vi "SQLite Get Sequence.vi"(8 "error in (no error)":errorcluster, 11 "Main":string="0") -> (0 "error out":errorcluster, 1 "TestMode List":string[](array[string]), 2 "GetRowHeaderList":string[](array[string]), 3 "TestSequence":string[][](array[string]), 4 "VariableName List":string[](array[string]))   [LabVIEW 2017, in "SQLite.lvclass"]
doc: "get test sequence table.\n2016-09-07 15:47:21\nBy：蒋松\nEmail：jiangsong@outlook.com\nSina: @sushu1051"
uses:
  SQLite.lvclass
  SQLiteFileName.ctl
  TabelFullName.ctl
  <vilib>/Utility/error.llb/Trim Whitespace.vi
  <userlib>/_OpenG.lib/array/array.llb/Remove Duplicates from 1D Array (String)__ogtk.vi
  <userlib>/LabSQL/LabSQL.lvlib
  <userlib>/sushu/sushu.lvlib
panel:
  out "Select SQL CMD":string
  out "Array 2":string[](array[string])
  out "Result Set":string[][](table) caption="Result Set (from first statement with results)"
  out "Array":string[](array[string])
  in  "SequenceNum":string
  in  "Items":string
  in  "Sequence Value":T1
  # "insert 之前要先backup原有的数据，使Items在对应条目的最大值+1\n2015-11-03 16:45:40\nBy：蒋松\nEmail：jiangsong@outlook.com\nSina: @sushu1051"
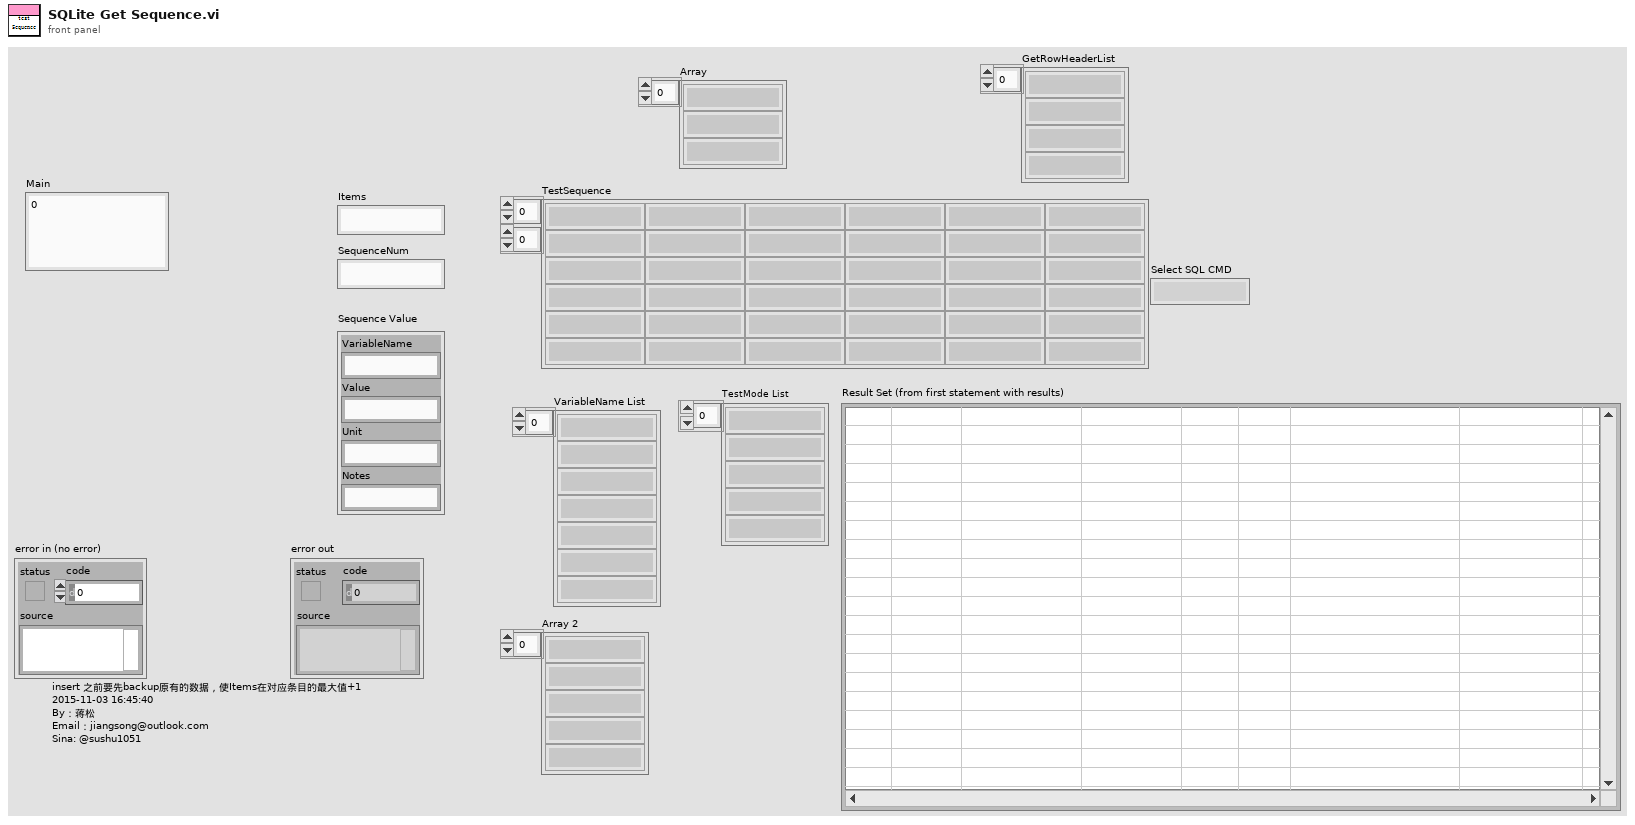
[diagram p1: front panel]
types:
  T1 = cluster{"VariableName":string, "Value":string, "Unit":string, "Notes":string}
  T2 = typedef "SQLite.lvclass/TabelFullName.ctl" = string
  T3 = typedef "SQLite.lvclass/SQLiteFileName.ctl" = string
  T4 = enum32{"invalid app kind", "Development System", "Run Time System", "Student Edition", "Embedded LabVIEW", "Evaluation", "Custom"}
  T5 = enum32{"Invalid", "Standard", "Closed", "Hidden", "Minimized", "Maximized"}
  T6 = enum16{"Other", "SQL2008", "SQLite", "Access", "MySQL"}
  T7 = cluster{"Core":cluster{"Current VI Reference":refnum<vi>, "Close Panel on Exit?":bool}}
  T8 = cluster{"Current VI Reference":refnum<vi>, "Close Panel on Exit?":bool}
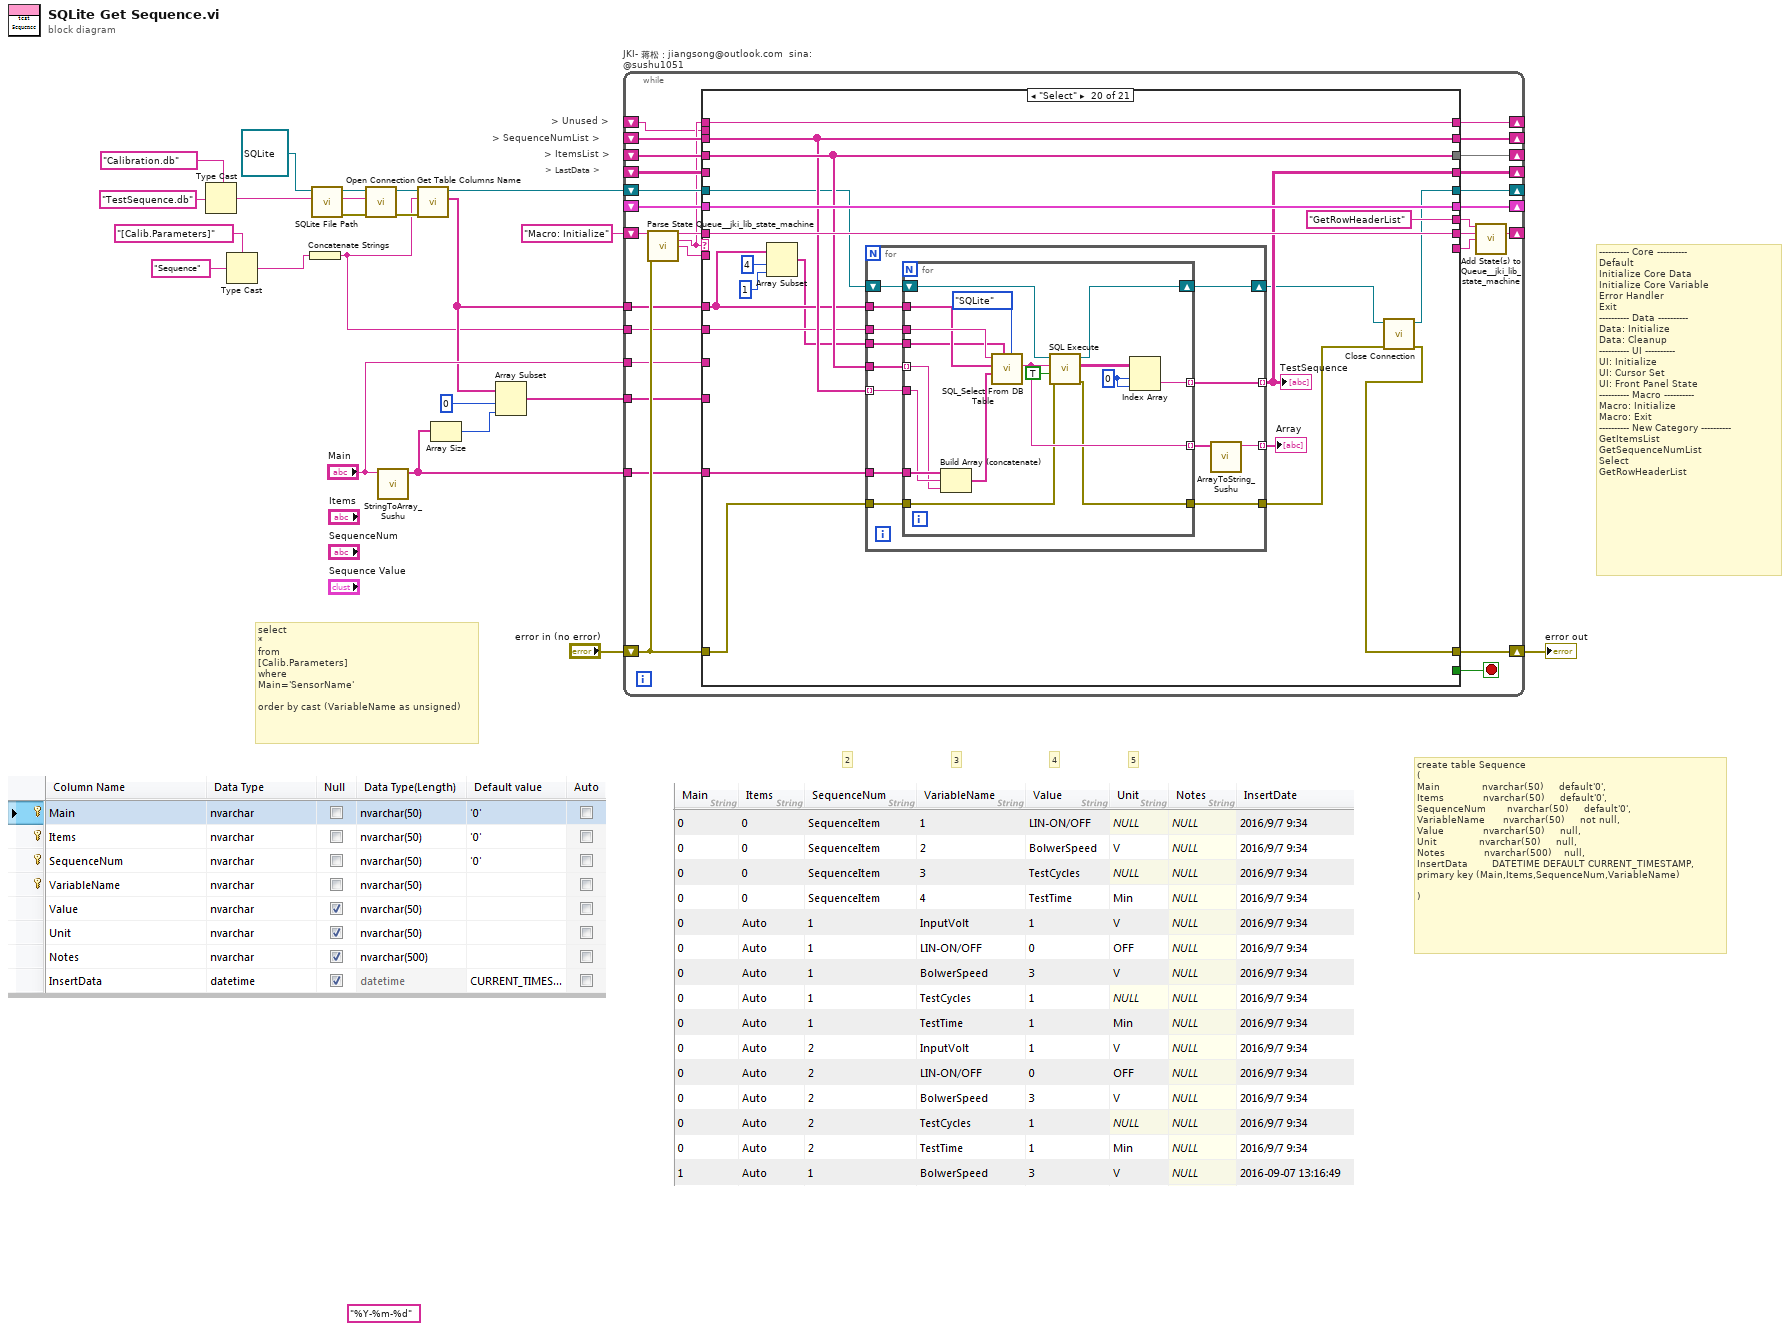
[diagram p0: block diagram]
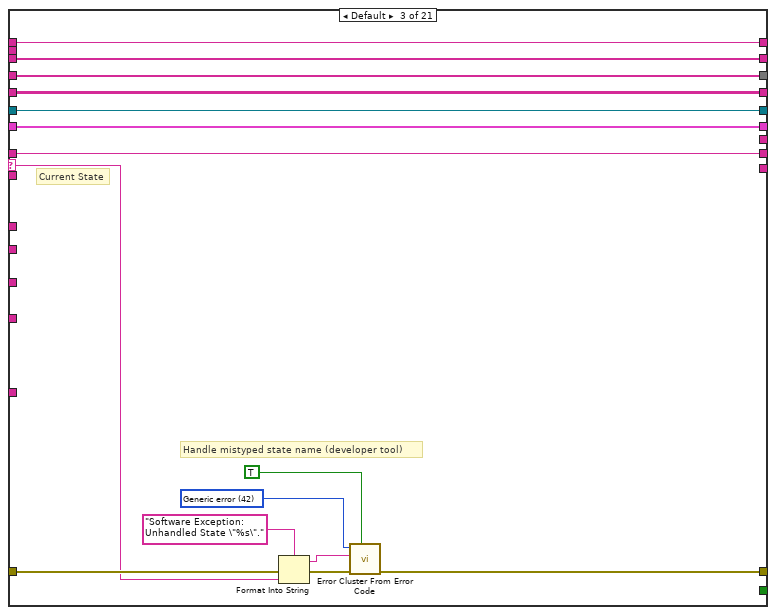
[diagram p4: hidden frame]
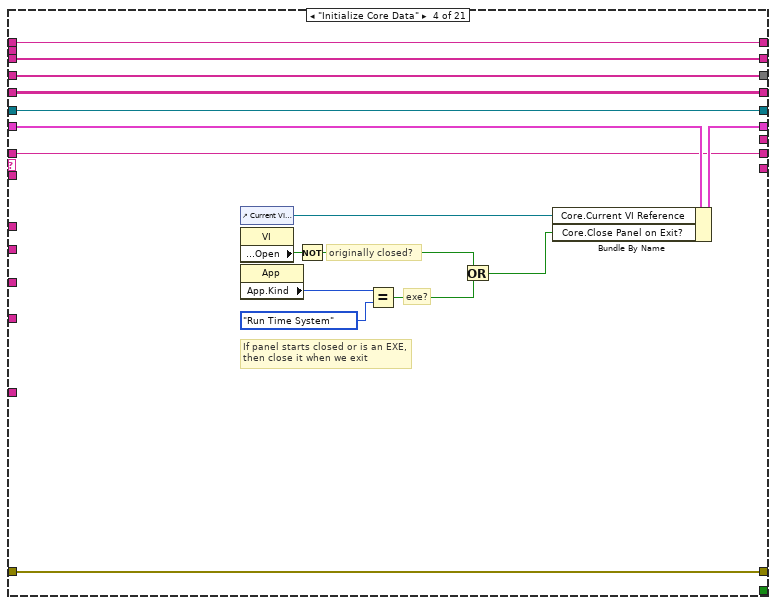
[diagram p5: hidden frame]
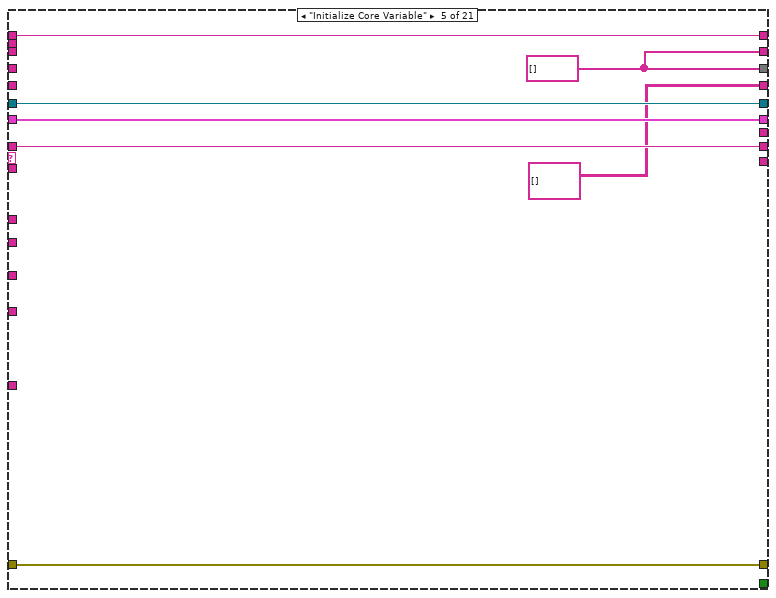
[diagram p6: hidden frame]
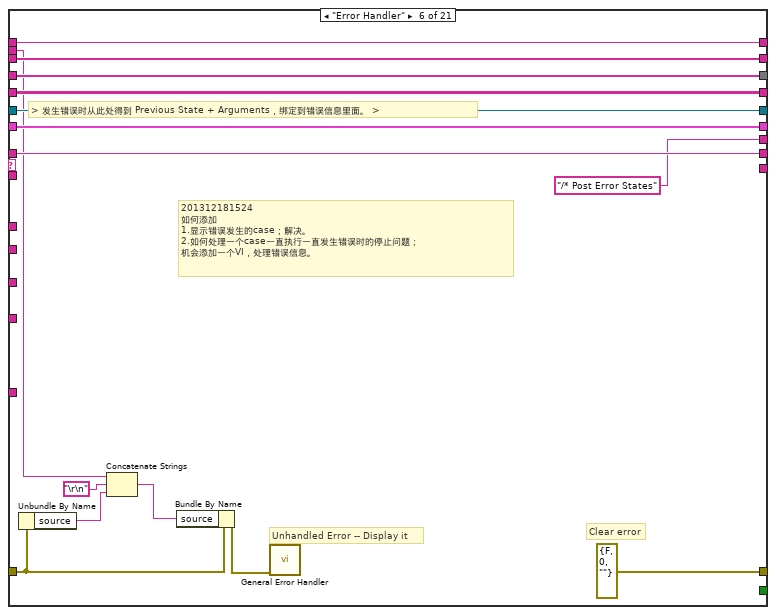
[diagram p7: hidden frame]
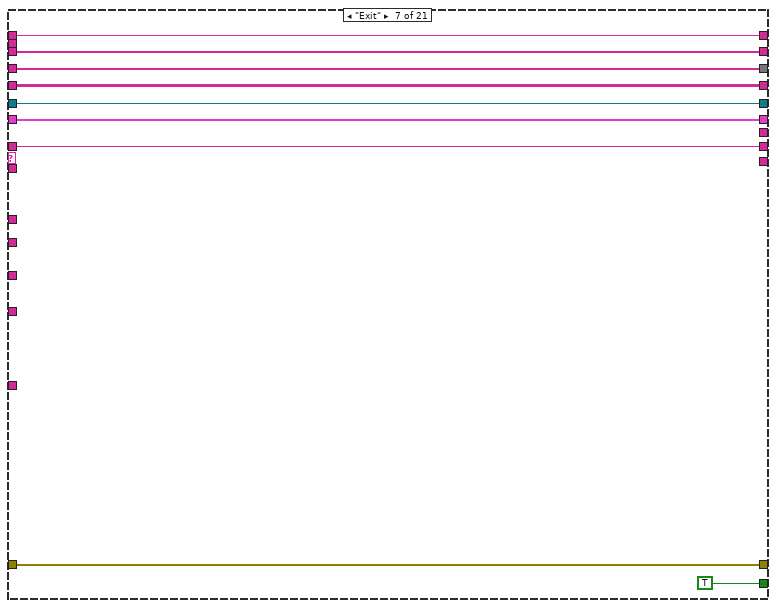
[diagram p8: hidden frame]
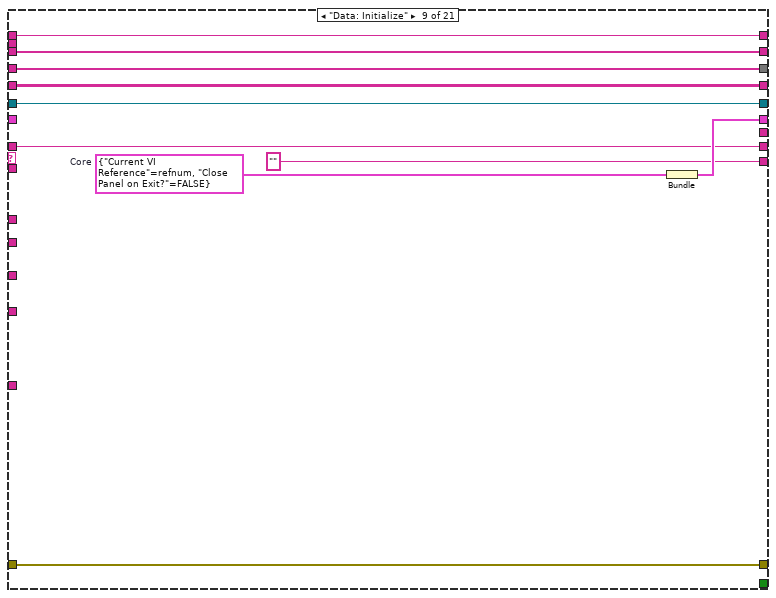
[diagram p10: hidden frame]
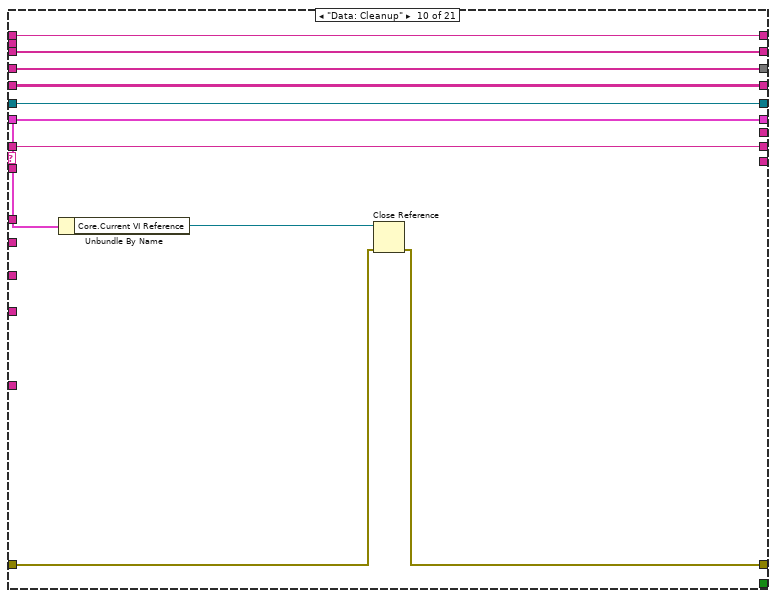
[diagram p11: hidden frame]
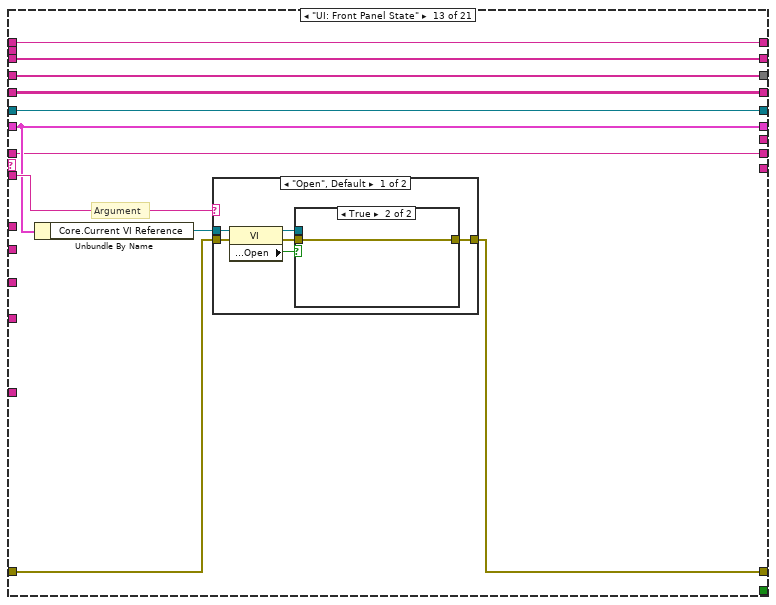
[diagram p14: hidden frame]
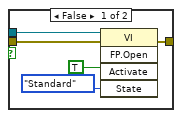
[diagram p15: hidden frame]
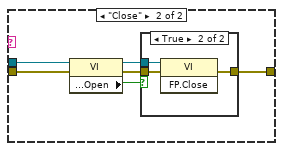
[diagram p16: hidden frame]
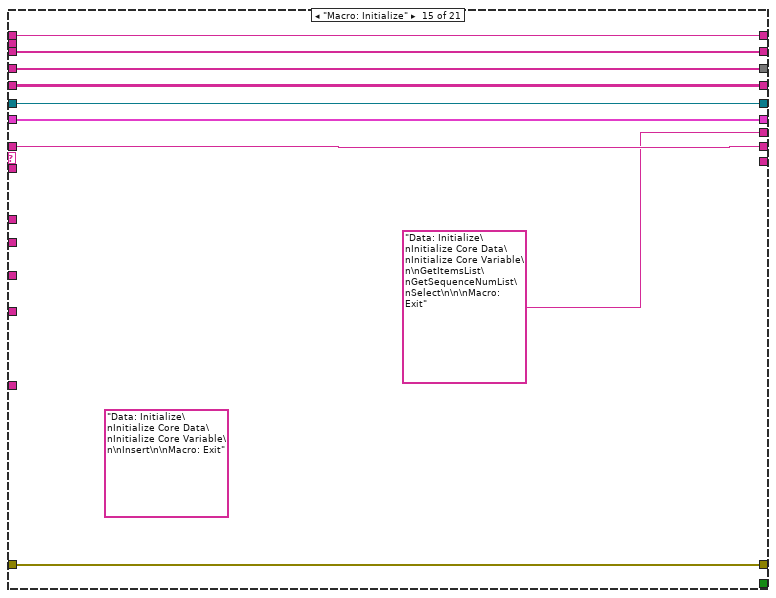
[diagram p19: hidden frame]
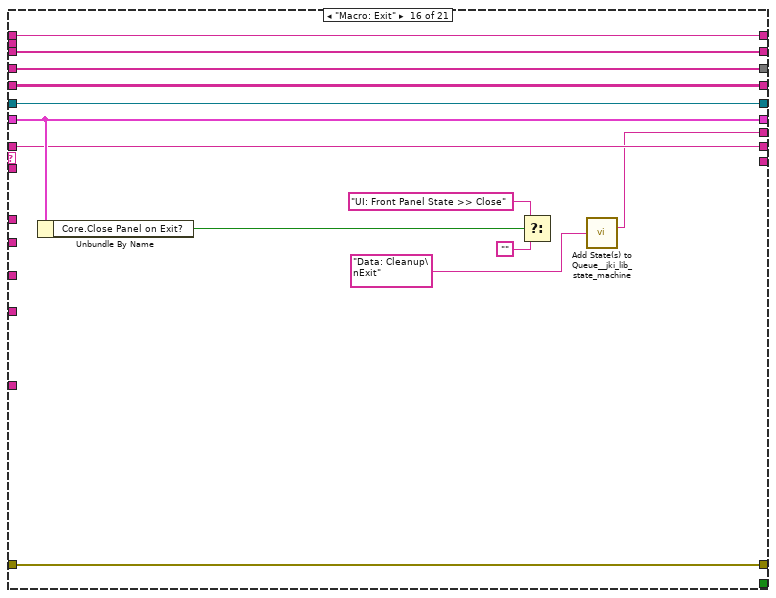
[diagram p20: hidden frame]
diagram:
  (unwired) "%Y-%m-%d" ("time format string (%c)")
  # "select\n*\nfrom\n[Calib.Parameters]\nwhere\nMain='SensorName'\n\norder by cast (VariableName as unsigned)"
  # "create table Sequence\n(\nMain              nvarchar(50)     default'0',\nItems             nvarchar(50)     default'0',\nSequenceNum       nvarchar(50)     default'0',\nVariableName      nvarchar(50)     not null,\nValue             nvarchar(50)     null,\nUnit              nvarchar(50)     null,\nNotes             nvarchar(500)    null,\nInsertData        DATETIME DEFAULT CURRENT_TIMESTAMP,\nprimary key (Main,Items,SequenceNum,VariableName)\n\n)"
  # "5"
  # "4"
  # "3"
  # "2"
  # "> Unused >"
  # "> LastData >"
  # "> ItemsList >"
  # "> SequenceNumList >"
  # "---------- Core ----------\nDefault\nInitialize Core Data\nInitialize Core Variable\nError Handler\nExit\n---------- Data ----------\nData: Initialize\nData: Cleanup\n---------- UI ----------\nUI: Initialize\nUI: Cursor Set\nUI: Front Panel State\n---------- Macro ----------\nMacro: Initialize\nMacro: Exit\n---------- New Category ----------\nGetItemsList\nGetSequenceNumList\nSelect\nGetRowHeaderList"
  n1 = Type Cast(type=T3 "Calibration.db" ("SQLiteFileName"), x="TestSequence.db" ("Remaining States")) -> (*(type *) &x=w12:T3)
  n2 = Type Cast(type=T2 "[Calib.Parameters]" ("TabelFullName"), x="Sequence" ("Remaining States")) -> (*(type *) &x=w15:T2)
  n3 = Concatenate Strings(w15) -> (w1:string)
  n4 = call "SQLite File Path.vi"("SQLiteFileName"=w12, "SQLite in"=refnum<class "SQLite.lvclass"> refnum ("SQLite.lvclass")) -> ("error out"=w9:errorcluster, "string"=w6:string, "SQLite out"=w8:refnum<class "SQLite.lvclass">)  [unwired: 7 in]
  n5 = call-dynamic "Open Connection.vi"("error in (no error)"=w9, "ConnectionString"=w6, "HostDB in"=w8) -> ("error out"=w5:errorcluster, "HostDB out"=w4:refnum<class "SQLite.lvclass">)  [unwired: 7 in]
  n6 = call <userlib>:"StringToArray_Sushu.vi"("State Queue"="Main") -> ("Array"=w18:string[])  [unwired: 8 in, 2 out]
  n7 = call-dynamic "Get Table Columns Name.vi"("error in (no error)"=w5, "TableName"=w1, "HostDB in"=w4) -> ("ColunmsList"=w2:string[], "HostDB out"=w3:refnum<class "SQLite.lvclass">)  [unwired: 4 in, 3 out]
  n8 = Array Size(array=w18) -> (size(s)=w17:i32)
  n9 = Array Subset(array=w2, index=0, length=w17) -> (w16:string[])
  n10 = while "JKI- 蒋松：jiangsong@outlook.com  sina: @sushu1051" {
    shift-right: [w49] -> w21
    shift-left: "error in (no error)" -> [w47]
    shift-right: [w36] -> _
    shift-left: "Macro: Initialize" -> [w37]
    shift-right: [w43] -> _
    shift-left: _ -> [w45]
    shift-right: [w44] -> _
    shift-left: _ -> [w46]
    shift-right: [w38] -> _
    shift-left: _ -> [w41]
    shift-right: [w39] -> _
    shift-left: w3 -> [w32]
    shift-right: [w40] -> _
    shift-left: _ -> [w42]
    shift-right: [w31] -> _
    shift-left: _ -> [w24]
    tunnel: w2 -> [w30]
    tunnel: w1 -> [w29]
    tunnel: "Main" -> [w28]
    tunnel: w18 -> [w27]
    tunnel: w16 -> [w26]
    stop <- w48 stop-if-true
    n11 = call <vilib>:"Parse State Queue__jki_lib_state_machine.vi"("State Queue"=w37, "Error In (no error)"=w47) -> ("Remaining States"=w51:string, "Current State"=w25:string, "Arguments"=w50:string)  [unwired: 10 in, 1 out]
    n12 = case shown="\"Select\"" w25 {
      selector: w25 -> [_ _ w70 _ _ _ _ _ _ _ _ _ _ _ _ _ _ _ _ _ _]
      tunnel: w51 -> [w59 w61 w69 w84 w103 w110 w122 w131 w140 w149 w159 w167 w175 w208 w217 w226 w238 w274 w306 w331 w371]
      tunnel: w50 -> [_ _ _ _ _ _ _ _ _ _ _ _ w178 _ _ _ _ _ _ _ _]
      tunnel: [w58 w67 w71 w95 w105 errorcluster {"status"=FALSE, "code"=0, "source"=""} ("error out") w124 w133 w144 w151 w161 w169 w179 w210 w219 w233 w241 w247 w277 w312 w372] -> w49
      tunnel: w47 -> [w58 w67 w72 w95 w105 w114 w124 w133 w144 w152 w161 w169 w180 w210 w219 w233 w241 w248 w278 w324 w372]
      tunnel: [w59 w61 w69 w84 w103 w110 w122 w131 w140 w149 w159 w167 w175 w208 w217 w226 w238 w274 w306 w331 w371] -> w35
      tunnel: [_ _ _ _ _ _ TRUE _ _ _ _ _ _ _ _ _ _ _ _ _ _] -> w48
      tunnel: w46 -> [w57 w66 w82 w98 _ w120 w129 w137 w147 w157 w165 w173 w184 w214 w223 w236 w244 w273 _ w327 w370]
      tunnel: w45 -> [w56 w65 w81 w97 _ w119 w128 w136 w146 w156 w164 w172 w183 w213 w222 w235 w243 _ w309 w328 w369]
      tunnel: [w57 w66 w82 w98 w100 w120 w129 w137 w147 w157 w165 w173 w184 w214 w223 w236 w244 w273 w293 w327 w370] -> w44
      tunnel: [w56 w65 w81 w97 w100 w119 w128 w136 w146 w156 w164 w172 w183 w213 w222 w235 w243 w254 w309 w328 w369] -> w43
      tunnel: w42 -> [w55 w64 w80 w96 _ w118 w127 w135 w145 w155 w163 w171 w182 w212 w221 w234 w242 w272 w308 _ w365]
      tunnel: w32 -> [w53 w62 w79 w85 w102 w108 w123 w132 w141 w150 w160 w168 w176 w209 w218 w227 w239 w252 w282 w318 w368]
      tunnel: w41 -> [w54 w63 w78 w87 w104 w117 w126 w134 _ w153 w162 w170 w177 w211 w220 w228 w240 w271 w307 w330 w367]
      tunnel: [w55 w64 w80 w96 string[][] [] ("Result Set") w118 w127 w135 w145 w155 w163 w171 w182 w212 w221 w234 w242 w272 w308 w317 w365] -> w40
      tunnel: [w53 w62 w79 w85 w102 w108 w123 w132 w141 w150 w160 w168 w176 w209 w218 w227 w239 w251 w281 w314 w368] -> w39
      tunnel: [w54 w63 w78 w86 w104 w117 w126 w134 w142 w153 w162 w170 w177 w211 w220 w228 w240 w271 w307 w330 w367] -> w38
      tunnel: [_ _ _ _ _ "/* Post Error States" _ _ _ _ _ _ _ _ "Data: Initialize\nInitialize Core Data\nInitialize Core Variable\n\nGetItemsList\nGetSequenceNumList\nSelect\n\n\nMacro: Exit" w225 _ _ _ "GetRowHeaderList" ("States Out") _] -> w34
      tunnel: [_ _ _ _ _ _ _ _ "" _ _ _ _ _ _ _ _ _ _ _ _] -> w33
      tunnel: w25 -> [w52 w60 w68 w83 w99 w107 w121 w130 w138 w148 w158 w166 w174 w207 w215 w224 w237 w270 w305 w329 w366]
      tunnel: [w52 w60 w68 w83 w99 w107 w121 w130 w138 w148 w158 w166 w174 w207 w215 w224 w237 w270 w305 w329 w366] -> w31
      tunnel: w30 -> [_ _ _ _ _ _ _ _ _ _ _ _ _ _ _ _ _ w258 w301 w323 _]
      tunnel: w29 -> [_ _ _ _ _ _ _ _ _ _ _ _ _ _ _ _ _ w268 w304 w326 _]
      tunnel: w28 -> [_ _ _ _ _ _ _ _ _ _ _ _ _ _ _ _ _ _ _ _ _]
      tunnel: w27 -> [_ _ _ _ _ _ _ _ _ _ _ _ _ _ _ _ _ _ w302 w325 _]
      tunnel: w26 -> [_ _ _ _ _ _ _ _ _ _ _ _ _ _ _ _ _ _ w303 _ _]
      tunnel: w24 -> [_ _ _ _ _ w106 _ _ _ _ _ _ _ _ _ _ _ _ _ _ _]
      frame "Idle" {
      }
      frame "---------- Core ----------" {
      }
      frame Default {
        w74 = 42 items=["No error", "Argument error", "Memory is full", "Out of zone", "End of file", "File already open", "Generic file I/O error", "File not found", "File permission error", "Disk is full", "Duplicate path", "Too many files open", "System feature not enabled", "Resource file not found", "Cannot add resource", "Resource not found", "Image not found", "Image memory error", "Pen does not exist", "Config type invalid", "Config token not found", "Config parse error", "Config memory error", "Bad external code format", "Bad external code offset", "External code not present", "Null window", "Destroy window error", "Null menu", "Print aborted", "Bad print record", "Print driver error", "Windows error during printing", "Memory error during printing", "Print dialog error", "Generic print error", "Invalid device refnum", "Device not found", "Device parameter error", "Device unit error", "Cannot open device", "Device call aborted", "Generic error", "Cancelled by user", "Object ID too low", "Object ID too high", "Object not in heap", "Unknown heap", "Unknown object (invalid DefProc)", "Unknown object (DefProc not in table)", "Message out of range", "Invalid (null) method", "Unknown message", "Manager call not supported", "Bad address", "Network operation in progress", "Network operation timed out", "Connection is busy", "Network attribute not supported", "Network error", "Address in use", "System out of memory", "Connection aborted", "Connection refused", "Not connected", "Already connected", "Connection closed", "Initialization error (interapplication manager)", "Bad occurrence", "Wait on unbound occurrence handler", "Occurrence queue overflow", "Datalog type conflict", "Unused", "Unrecognized type (interapplication manager)", "Memory corrupt", "Failed to make temporary DLL", "Old CIN version", "Drag socket not found", "Failed to load drop-object", "Failed to register OLE object", "Failed to release OLE object", "Format specifier type mismatch", "Unknown format specifier", "Too few format specifiers", "Too many format specifiers", "Scan failed", "Newer CIN version", "Error converting to variant", "Runtime menu error", "Password tampered", "Variant attribute not found", "Incompatible variant data type", "Event data is not available", "Event Store is not present", "Occurrence is not found", "Event Queue is not created", "Event info is not available", "Refnum passed is NULL", "Error retrieving Class GUID", "Error retrieving CoClass GUID", "Error retrieving TypeLib GUID.", "Bad built application magic bytes.", "Specific driver is different from the specific driver associated with the Logical Name.", "There is no session opened to the class driver.", "Max Error", "MAX - Error with config objects", "MAX - Error loading configuration", "MAX - Group not supported"]
        # "Current State"
        # "Handle mistyped state name (developer tool)"
        n13 = Format Into String(format string="Software Exception: Unhandled State \"%s\"." ("message"), error in=w72, w70) -> (resulting string=w75:string, error out=w76:errorcluster)  [unwired: 1 in]
        n14 = call <vilib>:"Error Cluster From Error Code.vi"("show call chain? (False)"=TRUE, "error in (no error)"=w76, "error message (\"\")"=w75, "error code (0)"=w74) -> ("error out"=w71:errorcluster)  [unwired: 5 in]
      }
      frame "Initialize Core Data" {
        # "originally closed?"
        # "exe?"
        # "If panel starts closed or is an EXE, then close it when we exit"
        n15 = control-ref of="Current VI Reference"() -> (w94:refnum<vi>)
        n16 = property class="VI"() -> ("Front Panel.Open"=w88:bool)  [unwired: 2 in, 2 out]
        n17 = property class="App"() -> ("App.Kind"=w89:T4)  [unwired: 2 in, 2 out]
        n18 = Not(x=w88) -> (.not. x?=w91:bool)
        n19 = Equal?(x=w89, y=T4."Run Time System" ("Application:Kind")) -> (x = y?=w92:bool)
        n20 = Or(x=w91, y=w92) -> (x .or. y?=w93:bool)
        n21 = Bundle By Name(cluster=w87, "Core.Current VI Reference"=w94, "Core.Close Panel on Exit?"=w93) -> (w86:T7)
      }
      frame "Initialize Core Variable" {
        w100 = string[] [] ("subarray")
      }
      frame "Error Handler" {
        # "> 发生错误时从此处得到 Previous State + Arguments，绑定到错误信息里面。 >"
        # "201312181524\n如何添加\n1.显示错误发生的case；解决。\n2.如何处理一个case一直执行一直发生错误时的停止问题；\n机会添加一个VI，处理错误信息。"
        # "Clear error"
        # "Unhandled Error -- Display it"
        n22 = Unbundle By Name(w114) -> ("source"=w112:string)
        n23 = Concatenate Strings(w106, "\r\n", w112) -> (w111:string)
        n24 = Bundle By Name(cluster=w114, "source"=w111) -> (w115:errorcluster)
        n25 = call <vilib>:"General Error Handler.vi"("error in (no error)"=w115) -> ()  [unwired: 10 in, 5 out]
      }
      frame "Exit" {
      }
      frame "---------- Data ----------" {
      }
      frame "Data: Initialize" {
        w143 = T8 {"Current VI Reference"=refnum, "Close Panel on Exit?"=FALSE}  # Core
        n26 = Bundle("Core"=w143) -> (w142:T7)  [unwired: 1 in]
      }
      frame "Data: Cleanup" {
        n27 = Unbundle By Name(w153) -> ("Core.Current VI Reference"=w154:refnum<vi>)
        n28 = Close Reference(reference=w154, error in (no error)=w152) -> (error out=w151:errorcluster)
      }
      frame "---------- UI ----------" {
      }
      frame "UI: Initialize" {
      }
      frame "UI: Front Panel State" {
        # "Argument"
        n29 = Unbundle By Name(w177) -> ("Core.Current VI Reference"=w181:refnum<vi>)
        n30 = case shown="\"Open\", Default" w178 {
          tunnel: w180 -> [w188 w201]
          tunnel: [w190 w202] -> w179
          tunnel: w181 -> [w189 w199]
          frame "Open", Default {
            n31 = property class="VI"(reference=w189, error in=w188) -> (reference out=w186:refnum<vi>, error out=w187:errorcluster, "Front Panel.Open"=w185:bool)
            n32 = case shown="True" w185 {
              tunnel: [w193 w196] -> w190
              tunnel: w187 -> [w192 w196]
              tunnel: w186 -> [w191 _]
              frame False {
                n33 = invoke class="VI" method="FP.Open"(reference=w191, error in=w192, "Activate"=TRUE, "State"=T5."Standard") -> (error out=w193:errorcluster)  [unwired: 1 in, 4 out]
              }
              frame True {
              }
            }
          }
          frame "Close" {
            n34 = property class="VI"(reference=w199, error in=w201) -> (reference out=w198:refnum<vi>, error out=w200:errorcluster, "Front Panel.Open"=w197:bool)
            n35 = case shown="True" w197 {
              tunnel: [w203 w206] -> w202
              tunnel: w200 -> [w203 w205]
              tunnel: w198 -> [_ w204]
              frame False {
              }
              frame True {
                n36 = invoke class="VI" method="FP.Close"(reference=w204, error in=w205) -> (error out=w206:errorcluster)  [unwired: 1 in, 2 out]
              }
            }
          }
        }
      }
      frame "---------- Macro ----------" {
      }
      frame "Macro: Initialize" {
        (unwired) "Data: Initialize\nInitialize Core Data\nInitialize Core Variable\n\nInsert\n\nMacro: Exit"
      }
      frame "Macro: Exit" {
        n37 = Unbundle By Name(w228) -> ("Core.Close Panel on Exit?"=w229:bool)
        n38 = Select(t="UI: Front Panel State >> Close", s=w229, f="") -> ()  [unwired: 1 out]
        n39 = call <vilib>:"Add State(s) to Queue__jki_lib_state_machine.vi"("State(s) at Back (\"\")"="Data: Cleanup\nExit") -> ("States Out"=w225:string)  [unwired: 14 in]
      }
      frame "---------- New Category ----------" {
      }
      frame "GetItemsList" {
        w260 = 3 ("length")
        # "string num >10 \nsequence not num list"
        n40 = Array Subset(array=w258, index=0, length=w260) -> (w266:string[])
        n41 = call <userlib>:"StringToArray_Sushu.vi"("State Queue"="0\n0\nSequenceItem" ("Main")) -> ("Array"=w265:string[])  [unwired: 8 in, 2 out]
        n42 = Index Array(array=w258, index=4) -> (element=w257:string)
        n43 = Index Array(array=w258, index=w260) -> (element=w261:string)
        n44 = Build Array(w257) -> (w253:string[])
        n45 = call <userlib>:"SQL_Select From DB Table.vi"("DB Type"=T6."SQLite", "SelectedColumnsNameList"=w253, "ColumnsValue"=w265, "ColumnsNameList"=w266, "TableName"=w268) -> ("Select SQL CMD"=w259:string)  [unwired: 6 in]
        n46 = Concatenate Strings(w259, "\r", "order by cast (" ("string"), w261, " as unsigned)" ("string")) -> (w250:string)
        n47 = call-dynamic "SQL Execute.vi"("error in (no error)"=w248, "Return Data (T)"=TRUE, "Command Text"=w250, "HostDB in"=w252) -> ("error out"=w247:errorcluster, "Table Control"=w249:string[][], "HostDB out"=w251:refnum<class "SQLite.lvclass">)  [unwired: 3 in, 2 out]
        n48 = Index Array(array=w249, index (col)=0 ("disabled index (col)")) -> (element=w254:string[])  [unwired: 1 in]
        "VariableName List" <- w254
      }
      frame "GetSequenceNumList" {
        w275 = T6."SQLite" ("DB Type")
        n49 = Index Array(array=w301, index=2) -> (element=w300:string)
        n50 = Build Array(w300) -> (w292:string[])
        n51 = call <userlib>:"SQL_Select From DB Table.vi"("DB Type"=w275, "ColumnsValue"=w302, "ColumnsNameList"=w303, "TableName"=w304) -> ("Select SQL CMD"=w288:string)  [unwired: 7 in]
        n52 = call <userlib>:"Build string_ColumnsName=ColumnsValue_Where and.vi"("DB Type"=w275, "=/!="="!=", "Have and?"=TRUE, "ColumnsValue"=string[] ["SequenceItem"], "Check ASCII?"=FALSE, "ColumnsNameList"=w292) -> ("ColumnName='ColumnValue'"=w289:string)  [unwired: 5 in]
        n53 = Concatenate Strings(w288, w289) -> (w280:string)
        "Select SQL CMD" <- w280
        n54 = call-dynamic "SQL Execute.vi"("error in (no error)"=w278, "Return Data (T)"=TRUE, "Command Text"=w280, "HostDB in"=w282) -> ("error out"=w277:errorcluster, "Table Control"=w279:string[][], "HostDB out"=w281:refnum<class "SQLite.lvclass">)  [unwired: 3 in, 2 out]
        "Result Set" <- w279
        n55 = Index Array(array=w279, index (col) #1=2 ("disabled index (col)"), index (col) #2=1 ("index (col)")) -> (element #1=w297:string[], element #2=w285:string[])  [unwired: 2 in]
        n56 = call-poly <userlib>:"Remove Duplicates from 1D Array__ogtk.vi"("Input Array"=w297) -> ("Output Array"=w296:string[])  [unwired: 1 out]
        n57 = call-poly <userlib>:"Remove Duplicates from 1D Array__ogtk.vi"("Input Array"=w285) -> ("Output Array"=→"TestMode List":string[])  [unwired: 1 out]
        n58 = Decimal String To Number(string=w296) -> (number=w295:i32[])  [unwired: 2 in, 1 out]
        n59 = Sort 1D Array(array=w295) -> (sorted array=w294:i32[])
        n60 = for {
          tunnel: w294 -> [w311] mode=indexing
          tunnel: [w310] -> w293 mode=indexing
          n61 = Number To Decimal String(number=w311) -> (decimal integer string=w310:string)  [unwired: 1 in]
        }
        "Array 2" <- w293
      }
      frame "Select" {
        n62 = Array Subset(array=w323, index=4, length=1) -> (w320:string[])
        n63 = for {
          tunnel: w328 -> [w344]
          tunnel: w327 -> [w339] mode=indexing
          shift-right: [w342] -> w315
          shift-left: w318 -> [w343]
          tunnel: w323 -> [w341]
          tunnel: w326 -> [w340]
          tunnel: w325 -> [w338]
          tunnel: w324 -> [w337]
          tunnel: [w336] -> w313
          tunnel: w320 -> [w335]
          tunnel: [w334] -> w319 mode=indexing
          tunnel: [w332] -> w317 mode=indexing
          n64 = for {
            tunnel: w344 -> [w358] mode=indexing
            shift-right: [w351] -> w342
            shift-left: w343 -> [w352]
            tunnel: w341 -> [w356]
            tunnel: w340 -> [w361]
            tunnel: w339 -> [w359]
            tunnel: w338 -> [w360]
            tunnel: w337 -> [w348]
            tunnel: [w347] -> w336
            tunnel: w335 -> [w355]
            tunnel: [w350] -> w333 mode=indexing
            tunnel: [w353] -> w332 mode=indexing
            w354 = 0 ("index (row)")
            n65 = Build Array (concatenate)(w360, w359, w358) -> (w357:string[])
            n66 = call <userlib>:"SQL_Select From DB Table.vi"("DB Type"=T6."SQLite", "SelectedColumnsNameList"=w355, "ColumnsValue"=w357, "ColumnsNameList"=w356, "TableName"=w361) -> ("Select SQL CMD"=w350:string)  [unwired: 6 in]
            n67 = call-dynamic "SQL Execute.vi"("error in (no error)"=w348, "Return Data (T)"=TRUE, "Command Text"=w350, "HostDB in"=w352) -> ("error out"=w347:errorcluster, "Table Control"=w349:string[][], "HostDB out"=w351:refnum<class "SQLite.lvclass">)  [unwired: 3 in, 2 out]
            n68 = Index Array(array=w349, index (row)=w354, index (col)=w354) -> (element=w353:string)
          }
          n69 = call <userlib>:"ArrayToString_Sushu.vi"("Array"=w333) -> ("String"=w334:string)  [unwired: 10 in]
        }
        "TestSequence" <- w317
        "Array" <- w319
        n70 = call-dynamic "Close Connection.vi"("error in (no error)"=w313, "HostDB in"=w315) -> ("error out"=w312:errorcluster, "HostDB out"=w314:refnum<class "SQLite.lvclass">)  [unwired: 8 in]
      }
      frame "GetRowHeaderList" {
        n71 = Array Size(array=w365) -> (size(s)=w364:i32[])
        n72 = Index Array(array=w364) -> (element=w363:i32)  [unwired: 1 in]
        n73 = for {
          N: w363 -> [_]
          tunnel: [w374] -> w362 mode=indexing
          i -> [w375]
          n74 = Increment(x=w375) -> (x+1=w373:i32)
          n75 = Number To Decimal String(number=w373) -> (decimal integer string=w374:string)  [unwired: 1 in]
        }
        "GetRowHeaderList" <- w362
      }
    }
    n76 = call <vilib>:"Add State(s) to Queue__jki_lib_state_machine.vi"("State(s) in Front (\"\")"=w34, "State(s) in (\"\")"=w35, "State(s) at Back (\"\")"=w33) -> ("States Out"=w36:string)  [unwired: 12 in]
  }
  "error out" <- w21
